vi "UI Refresh Data.vi"(8 "error in (no error)":errorcluster, 11 "Resource View in":refnum<class "Resource View.lvclass">) -> (0 "error out":errorcluster, 3 "Resource View out":refnum<class "Resource View.lvclass">)   [LabVIEW 2013, in "SET Project Editor.lvlib" / "Resource View.lvclass"]
uses:
  Resource View.lvclass
  UI View/UI View.lvclass/UI View.ctl
  SET Project Data/Project Data Class/Project Data.lvclass
  Resource View.lvclass/Resource View.ctl
  SET Project Data/Resource Data Class/Resource Data.lvclass/Resource Data.ctl
  UI View/Read _LangData.vi
  SET Project Data/Resource Data Class/Read Shared Resources.vi
  SET Project Data/Resource Data Class/Read Languages.vi
  SET Project Data/Resource Data Class/Resource Data.lvclass
panel:
  # "Trigger refresh of view's data"
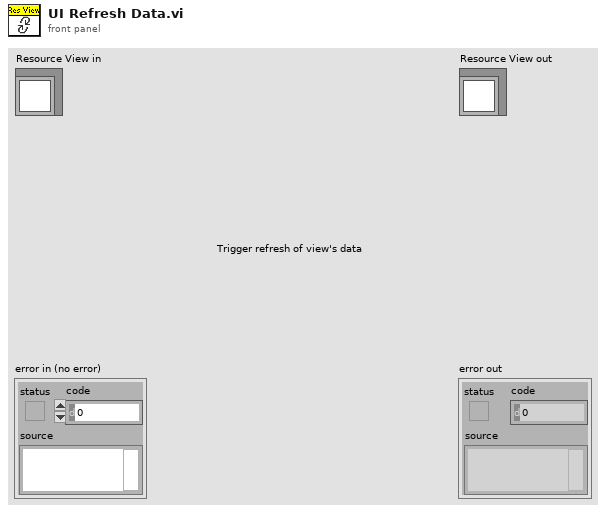
[diagram p1: front panel]
types:
  T1 = typedef "SET Project Data.lvlib/ProjFile_Resource Data.ctl" = cluster{"RID":string, "Tag":string, "Strings [] (UTF-16)":string[], "Shared?":bool}
  T2 = typedef "SET Project Data.lvlib/ProjFile_Language Data.ctl" = cluster{"Tag":string, "Name":string, "Code Page":u16}
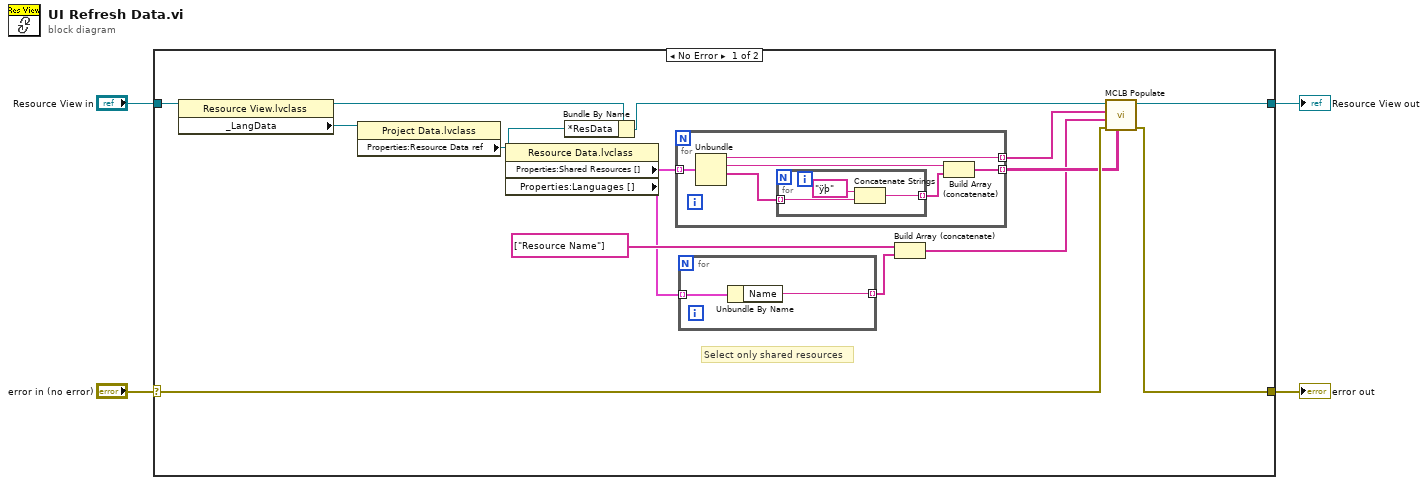
[diagram p0: block diagram]
diagram:
  n1 = case shown="No Error" "error in (no error)" {
    selector: "error in (no error)" -> [w15 w32]
    tunnel: "Resource View in" -> [w19 w31]
    tunnel: [w13 w31] -> w2
    tunnel: [w14 w32] -> w1
    frame No Error {
      # "Select only shared resources"
      n2 = property class="Resource View.lvclass"(reference=w19) -> (reference out=w9:refnum<class "Resource View.lvclass">, "_LangData"=w18:refnum<data-value>)  [unwired: 1 in, 1 out]
      n3 = property class="Project Data.lvclass"(reference=w18) -> ("Properties:Resource Data ref"=w7:refnum<data-value>)  [unwired: 1 in, 2 out]
      n4 = property class="Resource Data.lvclass"(reference=w7) -> ("Properties:Shared Resources []"=w16:T1[], "Properties:Languages []"=w6:T2[])  [unwired: 1 in, 2 out]
      n5 = Bundle By Name(cluster=w9, "*ResData"=w7) -> (w8:refnum<class "Resource View.lvclass">)
      n6 = for {
        tunnel: w16 -> [w27] mode=indexing
        tunnel: [w22] -> w12 mode=indexing
        tunnel: [w23] -> w11 mode=indexing
        n7 = Unbundle(w27) -> ("RID"=w23:string, "Tag"=w25:string, "Strings [] (UTF-16)"=w26:string[])  [unwired: 1 out]
        n8 = for {
          tunnel: w26 -> [w30] mode=indexing
          tunnel: [w28] -> w24 mode=indexing
          n9 = Concatenate Strings("ÿþ" ("string"), w30) -> (w28:string)
        }
        n10 = Build Array (concatenate)(w25, w24) -> (w22:string[])
      }
      n11 = for {
        tunnel: w6 -> [w21] mode=indexing
        tunnel: [w20] -> w5 mode=indexing
        n12 = Unbundle By Name(w21) -> ("Name"=w20:string)
      }
      n13 = Build Array (concatenate)(string[] ["Resource Name"], w5) -> (w10:string[])
      n14 = call-dynamic "MCLB Populate.vi"("Item Names[][]"=w12, "error in (no error)"=w15, "Column Header Strings[]"=w10, "Row Header Strings[]"=w11, "View in"=w8) -> ("error out"=w14:errorcluster, "View out"=w13:refnum<class "Resource View.lvclass">)  [unwired: 5 in]
    }
    frame Error {
    }
  }
  "error out" <- w1
  "Resource View out" <- w2
